vi "Start_trigger.vi"(8 "Error_in":errorcluster, 11 "VISA_in":refnum<visa-resource-name>) -> (0 "Error_out":errorcluster, 3 "VISA_out":refnum<visa-resource-name>)   [LabVIEW 2019]
uses:
  Measurement_Param_Global_Var.vi
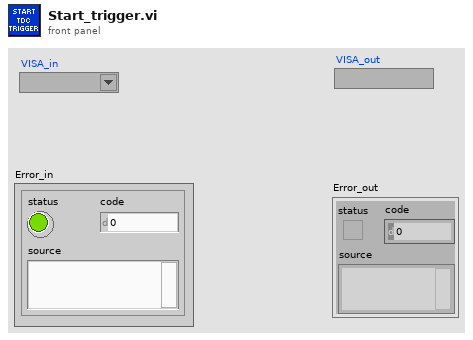
[diagram p1: front panel]
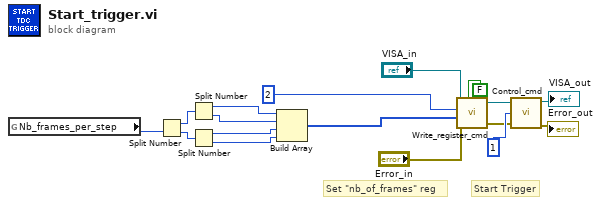
[diagram p0: block diagram]
diagram:
  # "Set \"nb_of_frames\" reg"
  # "Start Trigger"
  n1 = global read "Measurement_Param_Global_Var.vi" "Nb_frames_per_step"() -> (w7:u32)
  n2 = Split Number(x=w7) -> (hi(x)=w6:u16, lo(x)=w5:u16)
  n3 = Split Number(x=w6) -> (hi(x)=w4:u8, lo(x)=w3:u8)
  n4 = Split Number(x=w5) -> (hi(x)=w2:u8, lo(x)=w1:u8)
  n5 = Build Array(w4, w3, w2, w1) -> (w13:u8[])
  n6 = call "Write_register_cmd.vi"("Fifo-mode En"=FALSE, "Arty-7 Error In"="Error_in", "Data Array"=w13, "WrReg Addr"=u8 2, "Arty-7 VISA In"="VISA_in") -> ("Arty-7 Error out"=w16:errorcluster, "Arty-7 VISA out"=w15:refnum<visa-resource-name>)  [unwired: 3 in, 2 out]
  n7 = call "Control_cmd.vi"("Arty-7 Error In"=w16, "Control Command"=u8 1, "Arty-7 VISA In"=w15) -> ("Arty-7 Error out"=→"Error_out":errorcluster, "Arty-7 VISA out"=→"VISA_out":refnum<visa-resource-name>)  [unwired: 2 in, 2 out]
